vi "SPI_CS.vi"(0 "Value":bool, 1 "MXP Port":enum16{"A", "B"}(ring), 2 "Device":enum16{"CAN", "ENC", "IMU1", "IMU2"}(ring)) -> ()   [LabVIEW 2019]
uses:
  <vilib>/eio/EIONode/EIONode.xnode
  <vilib>/rvi/eio/common/nirviEmuTemplateMethod_errors.vi
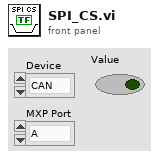
[diagram p1: front panel]
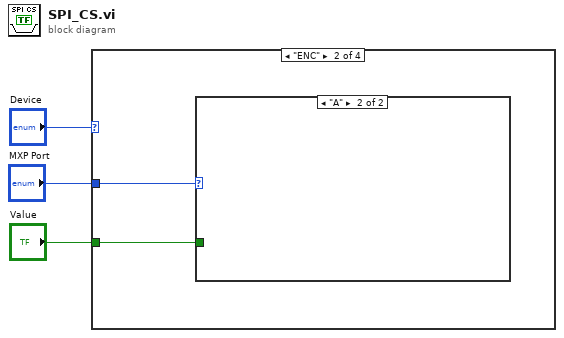
[diagram p0: block diagram]
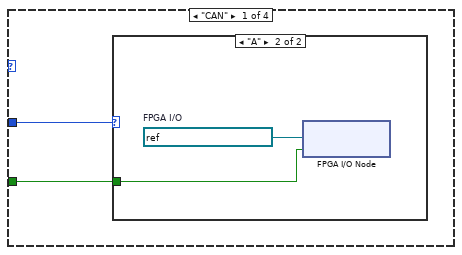
[diagram p2: hidden frame]
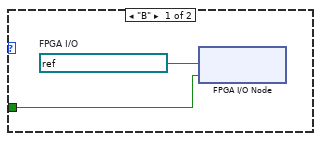
[diagram p3: hidden frame]
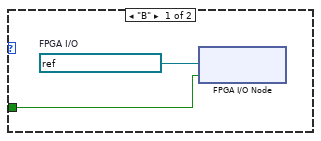
[diagram p4: hidden frame]
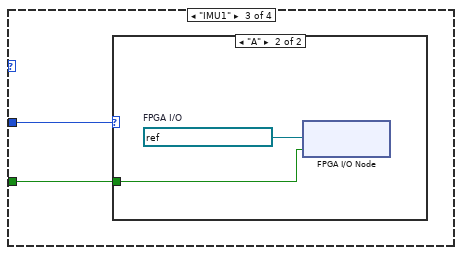
[diagram p5: hidden frame]
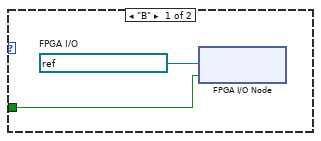
[diagram p6: hidden frame]
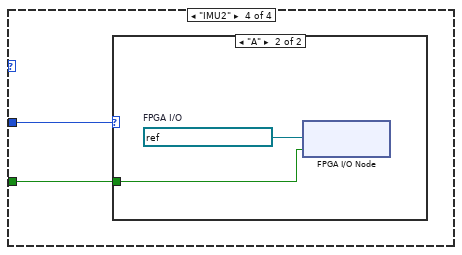
[diagram p7: hidden frame]
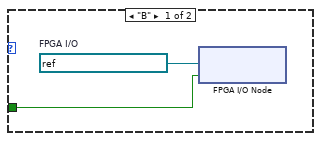
[diagram p8: hidden frame]
diagram:
  n1 = case shown="\"ENC\"" "Device" {
    tunnel: "MXP Port" -> [w5 w11 w16 w22]
    tunnel: "Value" -> [w4 w10 w15 w21]
    frame "CAN" {
      n2 = case shown="\"A\"" w5 {
        tunnel: w4 -> [w6 w8]
        frame "B" {
          w7 = refnum<k21> "ConnectorB/DIO13"  # FPGA I/O
          n3 = xnode "FPGA I/O Node"("I/O Item"=w6, "FPGA I/O In"=w7) -> ()  [unwired: 1 out]
        }
        frame "A" {
          w9 = refnum<k21> "ConnectorA/DIO13"  # FPGA I/O
          n4 = xnode "FPGA I/O Node"("I/O Item"=w8, "FPGA I/O In"=w9) -> ()  [unwired: 1 out]
        }
      }
    }
    frame "ENC" {
      n5 = case shown="\"A\"" w11 {
        tunnel: w10 -> [w12 w14]
        frame "B" {
          w13 = refnum<k21> "ConnectorB/DIO0"  # FPGA I/O
          n6 = xnode "FPGA I/O Node"("I/O Item"=w12, "FPGA I/O In"=w13) -> ()  [unwired: 1 out]
        }
        frame "A" {
        }
      }
    }
    frame "IMU1" {
      n7 = case shown="\"A\"" w16 {
        tunnel: w15 -> [w17 w19]
        frame "B" {
          w18 = refnum<k21> "ConnectorB/DIO12"  # FPGA I/O
          n8 = xnode "FPGA I/O Node"("I/O Item"=w17, "FPGA I/O In"=w18) -> ()  [unwired: 1 out]
        }
        frame "A" {
          w20 = refnum<k21> "ConnectorA/DIO12"  # FPGA I/O
          n9 = xnode "FPGA I/O Node"("I/O Item"=w19, "FPGA I/O In"=w20) -> ()  [unwired: 1 out]
        }
      }
    }
    frame "IMU2" {
      n10 = case shown="\"A\"" w22 {
        tunnel: w21 -> [w23 w25]
        frame "B" {
          w24 = refnum<k21> "ConnectorB/DIO11"  # FPGA I/O
          n11 = xnode "FPGA I/O Node"("I/O Item"=w23, "FPGA I/O In"=w24) -> ()  [unwired: 1 out]
        }
        frame "A" {
          w26 = refnum<k21> "ConnectorA/DIO11"  # FPGA I/O
          n12 = xnode "FPGA I/O Node"("I/O Item"=w25, "FPGA I/O In"=w26) -> ()  [unwired: 1 out]
        }
      }
    }
  }
